vi "MotorTest.vi"() -> ()   [LabVIEW 2020]
uses:
  <vilib>/Rock Robotics/SystemInterfaces/DIO/FPGA_DIOPWMChannel.ctl
  <vilib>/Rock Robotics/WPI/PWM/WPI_PWMDeadband.ctl
  <vilib>/Rock Robotics/WPI/MotorControl/WPI_MotorControlType.ctl
  <vilib>/Rock Robotics/SystemInterfaces/DIO/FPGA_DIOChannel.ctl
  <vilib>/Rock Robotics/WPI/MotorControl/WPI_MotorControlDeviceRef.ctl
panel:
  out "Right Lead Ref":T1={"DeviceStatus"={"status"=FALSE, "code"=0, "source"=""}, "Type"=enum."PWM", "PWM"={"PWM Channel"=enum."Invalid", "DeadBand"={"Name"="", "maxPositivePwm"=0, "minPositivePwm"=0, "centerPwm"=0, "maxNegativePwm"=0, "minNegativePwm"=0, "angularRange"=0}}, "CAN"={"Device Number"=0, "SetOutput VI Ref"=variant, "GetOutput VI Ref"=variant, "Enable VI Ref"=variant, "Disable VI Ref"=variant, "Data"=variant}, "Invert"=FALSE, "DIO PWM"={"PWM \"Enable\" Channel"=enum."Invalid", "DIOChannel"=enum."Invalid", "PWM Rate"=0.0}}
  out "error out":errorcluster
  out "Left Lead Ref":T1={"DeviceStatus"={"status"=FALSE, "code"=0, "source"=""}, "Type"=enum."PWM", "PWM"={"PWM Channel"=enum."Invalid", "DeadBand"={"Name"="", "maxPositivePwm"=0, "minPositivePwm"=0, "centerPwm"=0, "maxNegativePwm"=0, "minNegativePwm"=0, "angularRange"=0}}, "CAN"={"Device Number"=0, "SetOutput VI Ref"=variant, "GetOutput VI Ref"=variant, "Enable VI Ref"=variant, "Disable VI Ref"=variant, "Data"=variant}, "Invert"=FALSE, "DIO PWM"={"PWM \"Enable\" Channel"=enum."Invalid", "DIOChannel"=enum."Invalid", "PWM Rate"=0.0}}
  in  "CAN ID Right Follower":u8=4
  in  "CAN ID Right Leader":u8=3
  in  "CAN ID Left Follower":u8=2
  in  "CAN ID Left Leader":u8=1
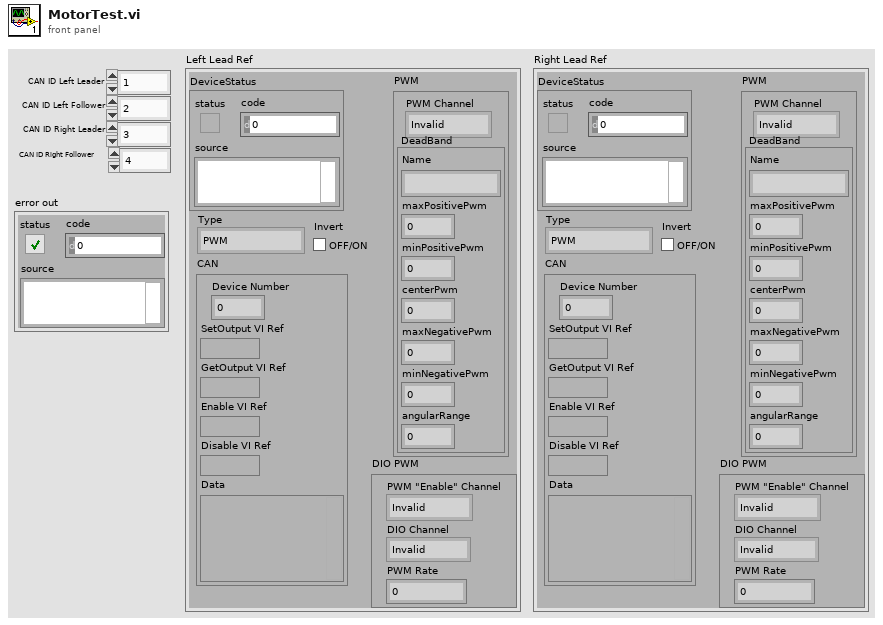
[diagram p1: front panel]
types:
  T1 = typedef "WPI_MotorControlDeviceRef.ctl" = cluster{"DeviceStatus":errorcluster, "Type":T2, "PWM":cluster{"PWM Channel":T3, "DeadBand":T4}, "CAN":cluster{"Device Number":u8, "SetOutput VI Ref":variant, "GetOutput VI Ref":variant, "Enable VI Ref":variant, "Disable VI Ref":variant, "Data":variant}, "Invert":bool, "DIO PWM":cluster{"PWM \"Enable\" Channel":T3, "DIOChannel":T5, "PWM Rate":dbl}}
  T2 = typedef "WPI_MotorControlType.ctl" = enum16{"PWM", "CAN", "DIO PWM"}
  T3 = typedef "FPGA_DIOPWMChannel.ctl" = enum8{"PWM 0", "PWM 1", "PWM 2", "PWM 3", "PWM 4", "PWM 5", "PWM 6", "PWM 7", "PWM 8", "PWM 9", "PWM MXP 0", "PWM MXP 1", "PWM MXP 2", "PWM MXP 3", "PWM MXP 4", "PWM MXP 5", "PWM MXP 6", "PWM MXP 7", "PWM MXP 8", "PWM MXP 9", "Invalid"}
  T4 = typedef "WPI_PWMDeadband.ctl" = cluster{"Name":string, "maxPositivePwm":i32, "minPositivePwm":i32, "centerPwm":i32, "maxNegativePwm":i32, "minNegativePwm":i32, "angularRange":u16}
  T5 = typedef "FPGA_DIOChannel.ctl" = enum8{"DIO 0", "DIO 1", "DIO 2", "DIO 3", "DIO 4", "DIO 5", "DIO 6", "DIO 7", "DIO 8", "DIO 9", "DIO MXP 0", "DIO MXP 1", "DIO MXP 2", "DIO MXP 3", "DIO MXP 4", "DIO MXP 5", "DIO MXP 6", "DIO MXP 7", "DIO MXP 8", "DIO MXP 9", "DIO MXP 10", "DIO MXP 11", "DIO MXP 12", "DIO MXP 13", "DIO MXP 14", "DIO MXP 15", "SPI Port CS1", "SPI Port CS2", "SPI Port CS3", "SPI Port MISO", "SPI Port MOSI", "Invalid"}
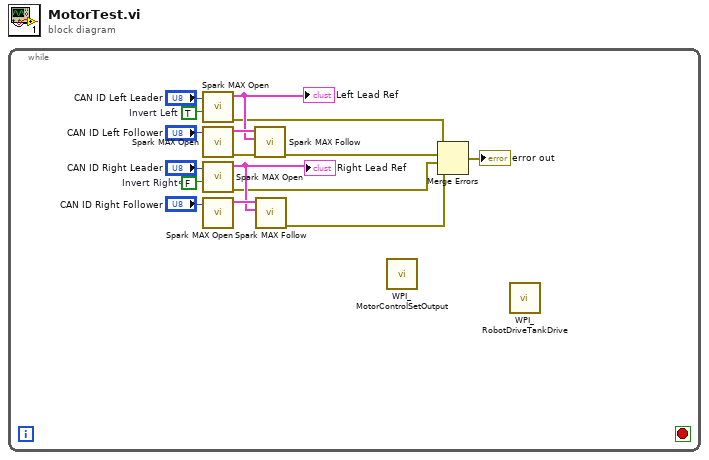
[diagram p0: block diagram]
diagram:
  n1 = while {
    stop <- _ stop-if-true
    w8 = TRUE  # Invert Left
    w9 = FALSE  # Invert Right
    n2 = call <vilib>:"Spark MAX Open.vi"("Invert"=w8, "Device Number"="CAN ID Left Leader") -> ("error out"=w5:errorcluster, "MotorControlDeviceRef"=w6:T1)  [unwired: 8 in]
    "Left Lead Ref" <- w6
    n3 = call <vilib>:"Spark MAX Open.vi"("Device Number"="CAN ID Left Follower") -> ("error out"=w13:errorcluster, "MotorControlDeviceRef"=w14:T1)  [unwired: 9 in]
    n4 = call <vilib>:"Spark MAX Open.vi"("Invert"=w9, "Device Number"="CAN ID Right Leader") -> ("error out"=w3:errorcluster, "MotorControlDeviceRef"=w7:T1)  [unwired: 8 in]
    "Right Lead Ref" <- w7
    n5 = call <vilib>:"Spark MAX Open.vi"("Device Number"="CAN ID Right Follower") -> ("MotorControlDeviceRef"=w12:T1)  [unwired: 9 in, 1 out]
    n6 = call <vilib>:"Spark MAX Follow.vi"("error in (no error)"=w13, "Master Controller"=w6, "MotorControlDeviceRef"=w14) -> ("error out"=w4:errorcluster)  [unwired: 7 in, 1 out]
    n7 = call <vilib>:"Spark MAX Follow.vi"("Master Controller"=w7, "MotorControlDeviceRef"=w12) -> ("error out"=w2:errorcluster)  [unwired: 8 in, 1 out]
    n8 = call <vilib>:"WPI_MotorControlSetOutput.vi"() -> ()  [unwired: 9 in, 3 out]
    n9 = Merge Errors(w5, w4, w3, w2) -> (→"error out":errorcluster)
    n10 = call <vilib>:"WPI_RobotDriveTankDrive.vi"() -> ()  [unwired: 9 in, 3 out]
  }
